vi "CheckRFLevel.vi"() -> ()   [LabVIEW 2025, in "Controls.lvlib"]
uses:
  Controls.lvlib
panel:
  out "RF Level OK":bool=TRUE
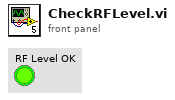
[diagram p1: front panel]
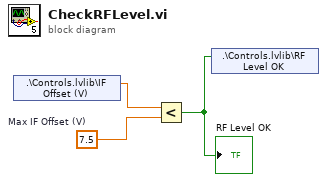
[diagram p0: block diagram]
diagram:
  w2 = 7.5  # Max IF Offset (V)
  n1 = shared-variable ".\\Controls.lvlib\\IF Offset (V)"() -> (w3:dbl)  [unwired: 1 in, 1 out]
  n2 = Less?(x=w3, y=w2) -> (x < y?=w1:bool)
  "RF Level OK" <- w1
  n3 = shared-variable ".\\Controls.lvlib\\RF Level OK"(w1) -> ()  [unwired: 1 in, 1 out]
